vi "SimpleRamp_Generate_FromTimeStep_v4.vi"(4 "error in (no error)":errorcluster, 5 "Error Locator":string, 6 "formula":string="sin(10*f)", 7 "Current Variable settings":T1[](array[typedef]), 8 "dt":dbl=1.0, 9 "TimeStep":dbl=500.0 min=0.0) -> (0 "error out":errorcluster, 1 "x values":dbl[](array[numeric]), 2 "y values":dbl[](array[numeric]), 3 "Remainder":dbl)   [LabVIEW 2013]
doc: "This VI computes a ramp where both the variable f and t are ramped. t is the total time from the start and f is the fraction of the total ramp time either may be used as a variable in the ramp equation.\n\nThis program takes a TimeStep which is the interval between points.\n\nThis program takes dt which is the total time of the ramp.\n\nThis returns the x and y values for the ramp and also the remainder time in case TimeStep didn't divide dt evenly."
uses:
  codes/TypeDefs/Active procedure variables.ctl
  NextMaster_v4.vi
  codes/PackedLibraries/LuaEvaluatorAPI.lvlibp
  SubVIs.lvlib
panel:
  # "This computes the expression, where\n\"f\" on the domain [0,1]\nor\n\"t\" varaible is in absolute units."
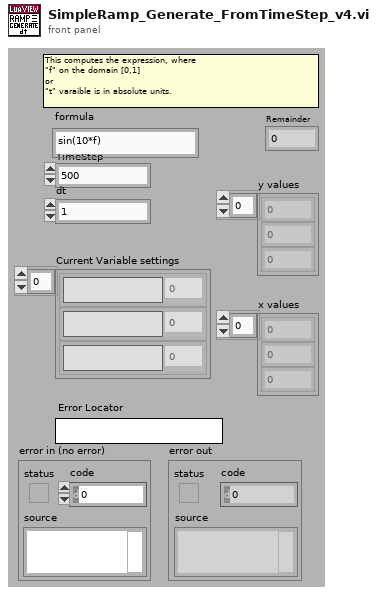
[diagram p1: front panel]
types:
  T1 = typedef "Active procedure variables.ctl" = cluster{"Procedure variable":string, "Value":dbl}
  T2 = enum16{"set", "get", "eval", "assign", "execute", "isvalid", "evaltable"}
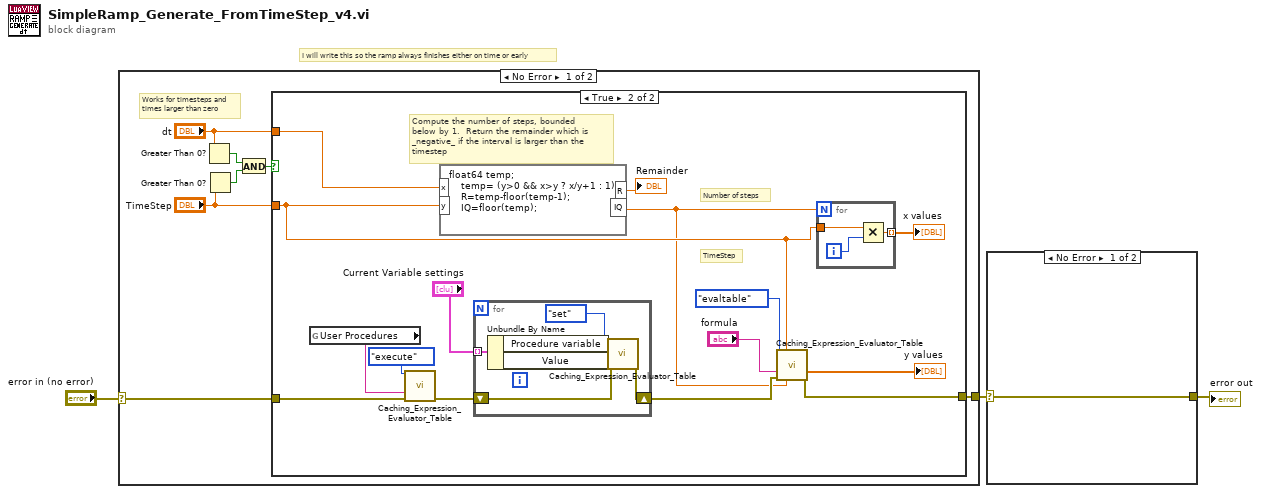
[diagram p0: block diagram]
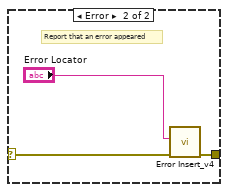
[diagram p2: hidden frame]
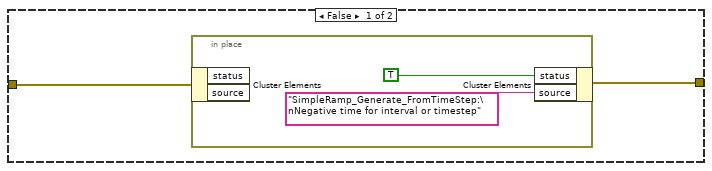
[diagram p3: hidden frame]
diagram:
  # "I will write this so the ramp always finishes either on time or early"
  n1 = case shown="No Error" "error in (no error)" {
    selector: "error in (no error)" -> [w9 w39]
    tunnel: [w10 w39] -> w1
    frame No Error {
      # "Works for timesteps and \ntimes larger than zero"
      n2 = Greater Than 0?(x="dt") -> (x > 0?=w5:bool)
      n3 = Greater Than 0?(x="TimeStep") -> (x > 0?=w4:bool)
      n4 = And(x=w5, y=w4) -> (x .and. y?=w6:bool)
      n5 = case shown="True" w6 {
        tunnel: [w11 w28] -> w10
        tunnel: w9 -> [w12 w21]
        tunnel: "dt" -> [_ w17]
        tunnel: "TimeStep" -> [_ w16]
        frame False {
          n6 = in-place {
            n7 = in-place-cluster #1(w12) -> ()  [unwired: 2 out]
            n8 = in-place-cluster #1("status"=TRUE, "source"="SimpleRamp_Generate_FromTimeStep:\nNegative time for interval or timestep") -> (w11:errorcluster)
          }
        }
        frame True {
          # "Compute the number of steps, bounded\nbelow by 1.  Return the remainder which is\n_negative_ if the interval is larger than the timestep"
          # "TimeStep"
          # "Number of steps"
          n9 = global read "NextMaster_v4.vi" "User Procedures"() -> (w20:string)
          n10 = call "Caching_Expression_Evaluator_Table.vi"("method"=T2."execute", "expression/scriptlet"=w20, "error in (no error)"=w21) -> ("error out"=w22:errorcluster)  [unwired: 4 in, 8 out]
          n11 = formula code="float64 temp;\n    temp= (y>0 && x>y ? x/y+1 : 1);\n    R=temp-floor(temp-1);\n    IQ=floor(temp);"("y"=w16, "x"=w17) -> ("R"=→"Remainder":dbl, "IQ"=w15:dbl)
          n12 = for {
            shift-right: [w38] -> w29
            shift-left: w22 -> [w37]
            tunnel: "Current Variable settings" -> [w34] mode=indexing
            n13 = Unbundle By Name(w34) -> ("Procedure variable"=w36:string, "Value"=w35:dbl)
            n14 = call "Caching_Expression_Evaluator_Table.vi"("method"=T2."set", "variable"=w36, "value in"=w35, "error in (no error)"=w37) -> ("error out"=w38:errorcluster)  [unwired: 3 in, 8 out]
          }
          n15 = call "Caching_Expression_Evaluator_Table.vi"("method"=T2."evaltable", "dt (for table)"=w16, "expression/scriptlet"="formula", "error in (no error)"=w29, "steps (for table)"=w15) -> ("table out"=→"y values":dbl[], "error out"=w28:errorcluster)  [unwired: 2 in, 7 out]
          n16 = for {
            N: w15 -> [_]
            tunnel: w16 -> [w32]
            tunnel: [w30] -> w25 mode=indexing
            i -> [w31]
            n17 = Multiply(x=w32, y=w31) -> (x*y=w30:dbl)
          }
          "x values" <- w25
        }
      }
    }
    frame Error {
    }
  }
  n18 = case shown="No Error" w1 {
    selector: w1 -> [w40 w43]
    tunnel: [w40 w42] -> w2
    frame No Error {
    }
    frame Error {
      # "Report that an error appeared"
      n19 = call "Error Insert_v4.vi"("error in (no error)"=w43, "error message (\"\")"="Error Locator") -> ("error out"=w42:errorcluster)  [unwired: 1 in, 6 out]
    }
  }
  "error out" <- w2
